vi "ADFX_About.vi"(0 "reference":refnum<vi>) -> ()   [LabVIEW 2015]
uses:
  <vilib>/XNodeSupport/NI_XNodeSupport.lvlib
panel:
  out "Version:":string
  # "Simple File Manager for the Adafruit Audio FX Sound Boards:\nhttps://learn.adafruit.com/adafruit-audio-fx-sound-board/overview\n\nGitHub: https://github.com/TangibleTec/Adafruit_FX_Programmer\n\nCompany:  TangibleTec, LLC (http://www.tangibletec.com)\nAuthor:       Ruben Kackstaetter\nLicense:      GPL 3"
  # "Click anywhere in this window to close."
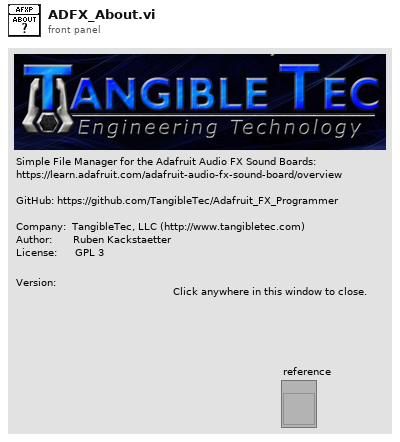
[diagram p1: front panel]
types:
  T1 = typedef "LVRectTypeDef.ctl" = cluster{"Left":i16, "Top":i16, "Right":i16, "Bottom":i16}
  T2 = typedef "NI_XNodeSupport.lvlib/XNodeBounds.ctl" = cluster{"Width":T3, "Height":T3}
  T3 = typedef "NI_XNodeSupport.lvlib/XNodeInt.ctl" = i32
  T4 = typedef "NI_XNodeSupport.lvlib/XNodeRect32.ctl" = cluster{"Left":T3, "Top":T3, "Right":T3, "Bottom":T3}
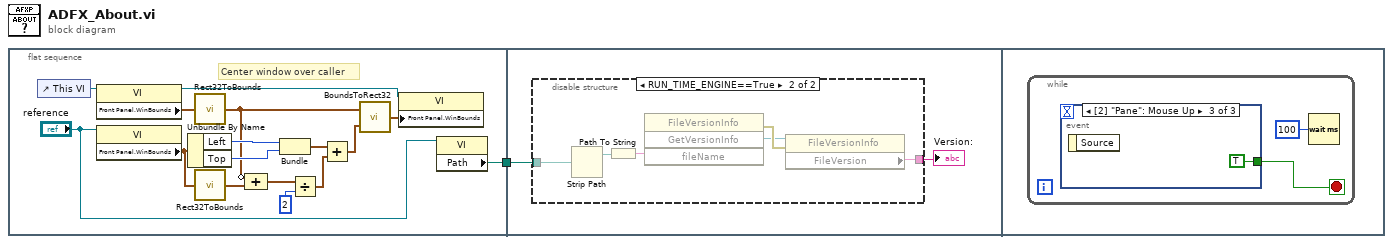
[diagram p0: block diagram]
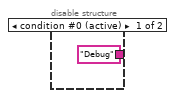
[diagram p2: hidden frame]
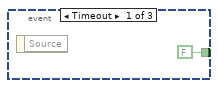
[diagram p3: hidden frame]
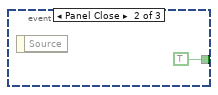
[diagram p4: hidden frame]
diagram:
  n1 = flat-sequence {
    tunnel: [w2] -> w1
    tunnel: w1 -> [w18]
    frame #0 {
      # "Center window over caller"
      n2 = control-ref of="This VI"() -> (w16:refnum<vi>)
      n3 = property class="VI"(reference=w16) -> (reference out=w17:refnum<vi>, "Front Panel.WinBounds"=w15:T1)  [unwired: 1 in, 1 out]
      n4 = property class="VI"(reference="reference") -> ("Front Panel.WinBounds"=w11:T1)  [unwired: 1 in, 2 out]
      n5 = Unbundle By Name(w11) -> ("Left"=w9:i16, "Top"=w10:i16)
      n6 = call <vilib>:"Rect32ToBounds.vi"("Rect32"=w15) -> ("Bounds"=w4:T2)
      n7 = call <vilib>:"Rect32ToBounds.vi"("Rect32"=w11) -> ("Bounds"=w5:T2)
      n8 = Compound Arithmetic op=ADD(invert w4, w5) -> (w13:T2)
      n9 = Bundle("Left"=w9, "Top"=w10) -> (w7:cluster{"Left":i16, "Top":i16})  [unwired: 1 out]
      n10 = Divide(x=w13, y=2) -> (x/y=w8:cluster{"Width":dbl, "Height":dbl})
      n11 = Add(x=w7, y=w8) -> (x+y=w6:cluster{dbl, dbl})
      n12 = call <vilib>:"BoundsToRect32.vi"("Offset (0,0)"=w6, "Bounds"=w4) -> ("Rect32"=w14:T4)
      n13 = property class="VI"(reference=w17, "Front Panel.WinBounds"=w14) -> ()  [unwired: 1 in, 2 out]
      n14 = property class="VI"(reference="reference") -> ("Path"=w2:path)  [unwired: 1 in, 2 out]
    }
    frame #1 {
      n15 = disable-structure shown="RUN_TIME_ENGINE==True" {
        disable-tunnel: ["Debug" ("Version of Executable") w22] -> w19
        disable-tunnel: w18 -> [_ w21]
        frame condition #0 (active) {
        }
        frame condition #1 {
          n16 = Strip Path(path=w21) -> (stripped path=w26:path)  [unwired: 1 out]
          n17 = Path To String(path=w26) -> (string=w23:string)
          n18 = invoke class="FileVersionInfo" method="GetVersionInfo"("fileName"=w23) -> (error out=w25:errorcluster, "GetVersionInfo"=w24:refnum<k24>)  [unwired: 3 in, 2 out]
          n19 = property class="FileVersionInfo"(reference=w24, error in=w25) -> ("FileVersion"=w22:string)  [unwired: 2 out]
        }
      }
      "Version:" <- w19
    }
    frame #2 {
      n20 = while {
        stop <- w27 stop-if-true
        n21 = event shown="[2] \"Pane\": Mouse Up" {
          selector: _ -> [_ _ _]
          dyn-events: _ -> [_ _ _]
          timeout: _ -> [_ _ _]
          tunnel: [FALSE TRUE TRUE] -> w27
          event Timeout {
            n22 = event-data() -> ()  [unwired: 1 in, 1 out]
          }
          event Panel Close {
            n23 = event-data() -> ()  [unwired: 1 in, 1 out]
          }
          event Mouse Up {
            n24 = event-data() -> ()  [unwired: 1 in, 1 out]
          }
        }
        n25 = Wait (ms)(milliseconds to wait=u32 100) -> ()  [unwired: 1 out]
      }
    }
  }
